vi "CRYSet Title Name and Icon from Type.vi"   [LabVIEW 2013]
uses:
  CRYWindow/SubVI/CRYMain Sub Window Global.vi
types:
  T1 = typedef "LVRectTypeDef.ctl" = cluster{"Left":i16, "Top":i16, "Right":i16, "Bottom":i16}
  T2 = cluster{"nID":i32[], "Frame":cluster{"nType":i32, "nParent":i32, "pVIW":refnum<vi>, "pSPW":refnum<vi>, "nTypeF":i32, "pVIF":refnum<vi>, "pSPF":refnum<vi>, "nIDSpliter":i32, "nProperty":i32, "Bound":T1, "nID":i32, "nData":i32, "sData":string, "pWVI":refnum<vi>, "sTitle":string, "cPages":cluster{"nPage":i32, "sTitle":string, "sIcon":string, "pVI":refnum<vi>, "nID":i32}[], "pTab":refnum<vi>, "nIDPages":i32[], "pSPT":refnum<vi>, "sTemp":string, "nDockID":i32, "nDockLR":i32, "sIcon":string}[]}
  T3 = cluster{"nType":i32, "nParent":i32, "pVIW":refnum<vi>, "pSPW":refnum<vi>, "nTypeF":i32, "pVIF":refnum<vi>, "pSPF":refnum<vi>, "nIDSpliter":i32, "nProperty":i32, "Bound":T1, "nID":i32, "nData":i32, "sData":string, "pWVI":refnum<vi>, "sTitle":string, "cPages":cluster{"nPage":i32, "sTitle":string, "sIcon":string, "pVI":refnum<vi>, "nID":i32}[], "pTab":refnum<vi>, "nIDPages":i32[], "pSPT":refnum<vi>, "sTemp":string, "nDockID":i32, "nDockLR":i32, "sIcon":string}[]
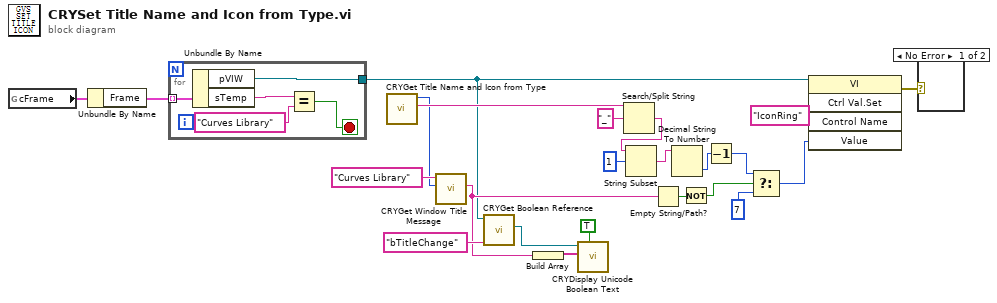
[diagram p0: block diagram]
diagram:
  n1 = global read "CRYMain Sub Window Global.vi" "cFrame"() -> (w9:T2)
  n2 = Unbundle By Name(w9) -> ("Frame"=w8:T3)
  n3 = for {
    tunnel: w8 -> [w28] mode=indexing
    tunnel: [w24] -> w2
    stop <- w25 stop-if-true
    n4 = Unbundle By Name(w28) -> ("pVIW"=w24:refnum<vi>, "sTemp"=w26:string)
    n5 = Equal?(x=w26, y="Curves Library" ("Kind")) -> (x = y?=w25:bool)
  }
  n6 = call "CRYGet Title Name and Icon from Type.vi"() -> ("Icon Name"=w12:string, "Title No"=w10:i32)  [unwired: 10 in]
  n7 = call "CRYGet Window Title Message.vi"("No"=w10, "Kind"="Curves Library") -> ("Unicode String"=w4:string)  [unwired: 4 in, 5 out]
  n8 = call "CRYGet Boolean Reference.vi"("Label Name"="bTitleChange" ("Control Name"), "VI Refnum"=w2) -> ("Boolean Ref"=w7:refnum<vi>)  [unwired: 7 in, 2 out]
  n9 = Build Array(w4) -> (w5:string[])
  n10 = call "CRYDisplay Unicode Boolean Text.vi"("Interpret as Unicode (T)"=TRUE, "Boolean Texts [4]"=w5, "Boolean Reference"=w7) -> ()  [unwired: 5 in, 2 out]
  n11 = Search/Split String(string=w12, search string/char (-)="_" ("search string")) -> (match + rest of string=w21:string)  [unwired: 3 out]
  n12 = String Subset(string=w21, offset (0)=1) -> (substring=w19:string)  [unwired: 1 out]
  n13 = Empty String/Path?(string/path=w4) -> (empty?=w16:bool)
  n14 = Decimal String To Number(string=w19) -> (number=w18:i32)  [unwired: 3 out]
  n15 = Not(x=w16) -> (.not. x?=w15:bool)
  n16 = Decrement(x=w18) -> (x-1=w17:i32)
  n17 = Select(t=w17, s=w15, f=7) -> (s? t:f=w13:i32)
  n18 = invoke class="VI" method="Ctrl Val.Set"(reference=w2, "Control Name"="IconRing", "Value"=w13) -> (error out=w1:errorcluster)  [unwired: 2 in, 4 out]
  n19 = case shown="No Error" w1 {
    frame No Error {
    }
    frame Error {
    }
  }
